vi "MTIF_Read_Simple.vi"(8 "error in":errorcluster, 9 "Input Parameters":T2={"Drop Bits"=3, "Output Files?"=TRUE, "STD Threshold Ratio for Start"=1.2, "STD Threshold Ratio for Stop"=1.1, "Output Image Type"=0, "Timeout for Queue(ms)"=1000, "Output Queue?"=FALSE, "Output File Format"=enum."AVI", "Initial STD Threshold"=12.0, "Number of Buffered Frames"=150, "Centroid Distence Threshold"=1.0} {"Output Image Type" items=["Grayscale (U8)", "Grayscale (I16)", "Grayscale (SGL)", "Complex (CSG)", "RGB (U32)", "HSL (U32)", "RGB (U64)", "Grayscale (U16)"]}, 10 "File Name (.mtif)":string="t8", 11 "Folder Path":path=path "X:/Zebrafish_VR_Data") -> (0 "error out":errorcluster, 2 "U8 Array Queue Out":refnum<queue>, 3 "U16 Array Queue Out":refnum<queue>)   [LabVIEW 2019]
uses:
  <vilib>/vision/NI_Vision_Development_Module.lvlib
panel:
  in  "Stop":bool
  out "Frame No.":i32=58
  out "Sequence No.":u16=3128
  out "Progress":dbl=1.0 format="%#.3f"
  out "Raw Image":T3(plugin-control)
  out "Frame Rate":dbl=550.0
  out "File ROI":T4={"Left"=0, "Top"=0, "Right"=639, "Bottom"=479, "Rotation"=0.0} {"Rotation" format="%.2f"; "Left" scale=0.0..1024.0; "Right" scale=0.0..1024.0}
  # "Max 2GB\nfor one AVI file!"
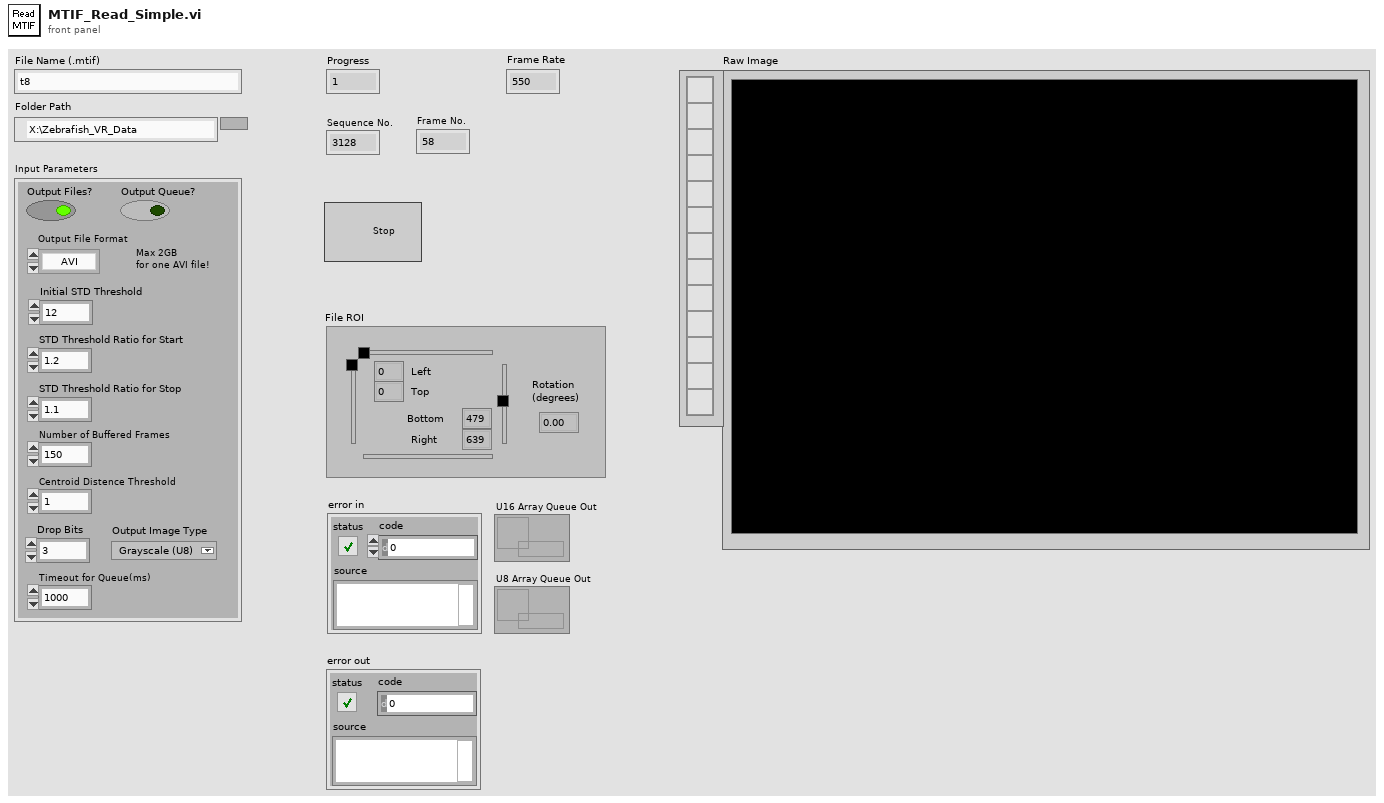
[diagram p1: front panel]
types:
  T1 = typedef "Image Type" = u32
  T2 = cluster{"Drop Bits":i8, "Output Files?":bool, "STD Threshold Ratio for Start":dbl, "STD Threshold Ratio for Stop":dbl, "Output Image Type":T1, "Timeout for Queue(ms)":u32, "Output Queue?":bool, "Output File Format":enum16{"TIFF", "AVI"}, "Initial STD Threshold":sgl, "Number of Buffered Frames":i32, "Centroid Distence Threshold":sgl}
  T3 = typedef "IMAQ Image.ctl" = refnum<image>
  T4 = typedef "IMAQ Rectangle" = cluster{"Left":i32, "Top":i32, "Right":i32, "Bottom":i32, "Rotation":dbl}
  T5 = enum16{"big-endian, network order", "native, host order", "little-endian"}
  T6 = enum16{"open", "replace", "create", "open or create", "replace or create", "replace or create with confirmation"}
  T7 = cluster{"[0]":i32, "[1]":i32, "[2]":i32, "[3]":i32}
  T8 = typedef "IMAQ AVI2 Refnum.ctl" = refnum<k20>
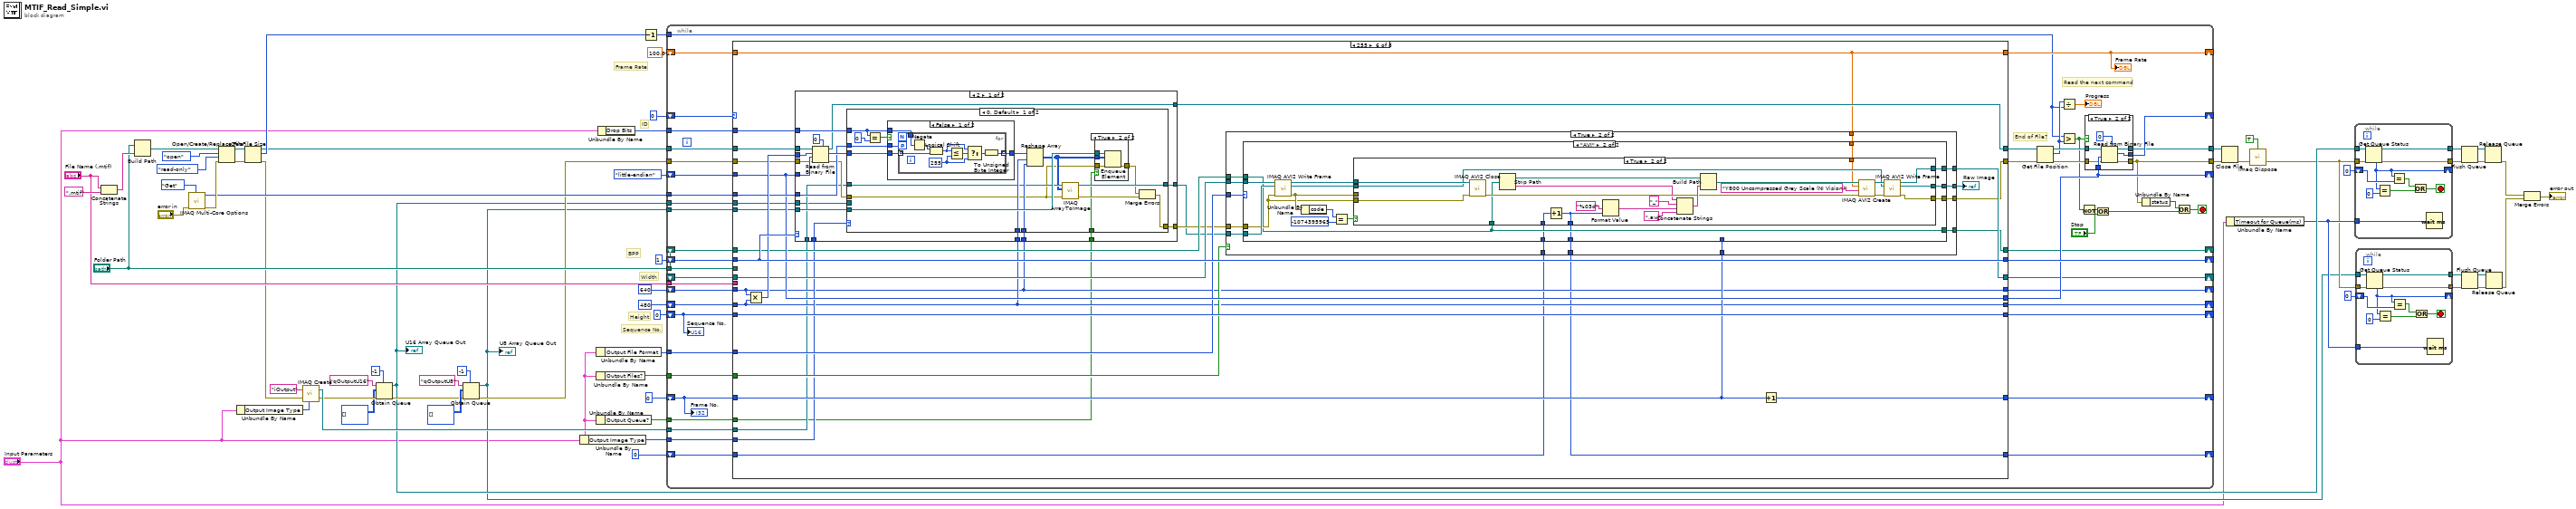
[diagram p0: block diagram]
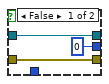
[diagram p2: hidden frame]
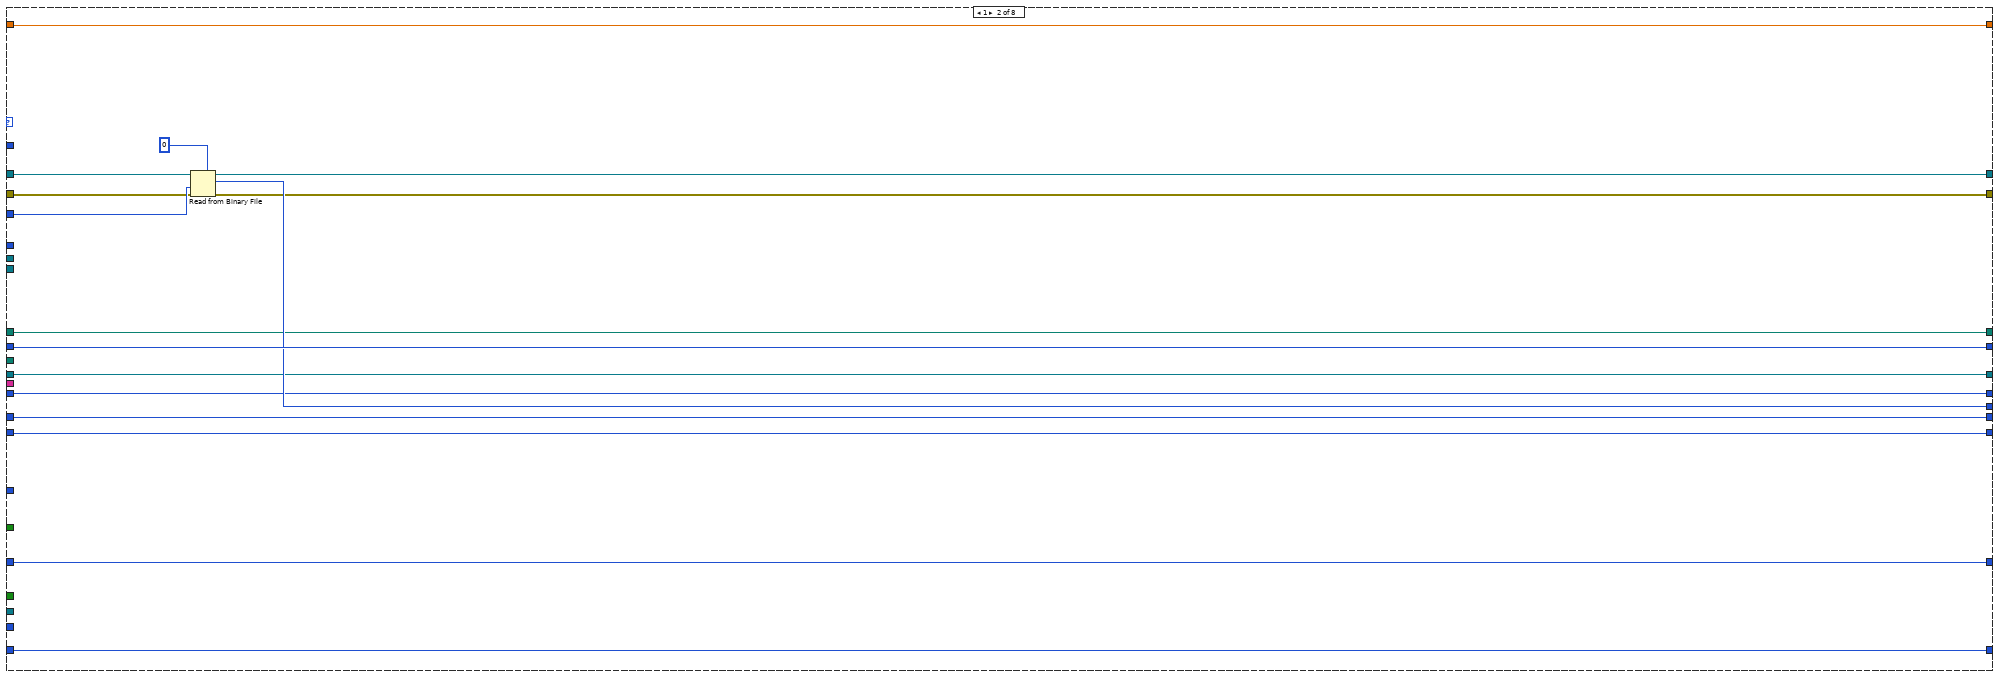
[diagram p4: hidden frame]
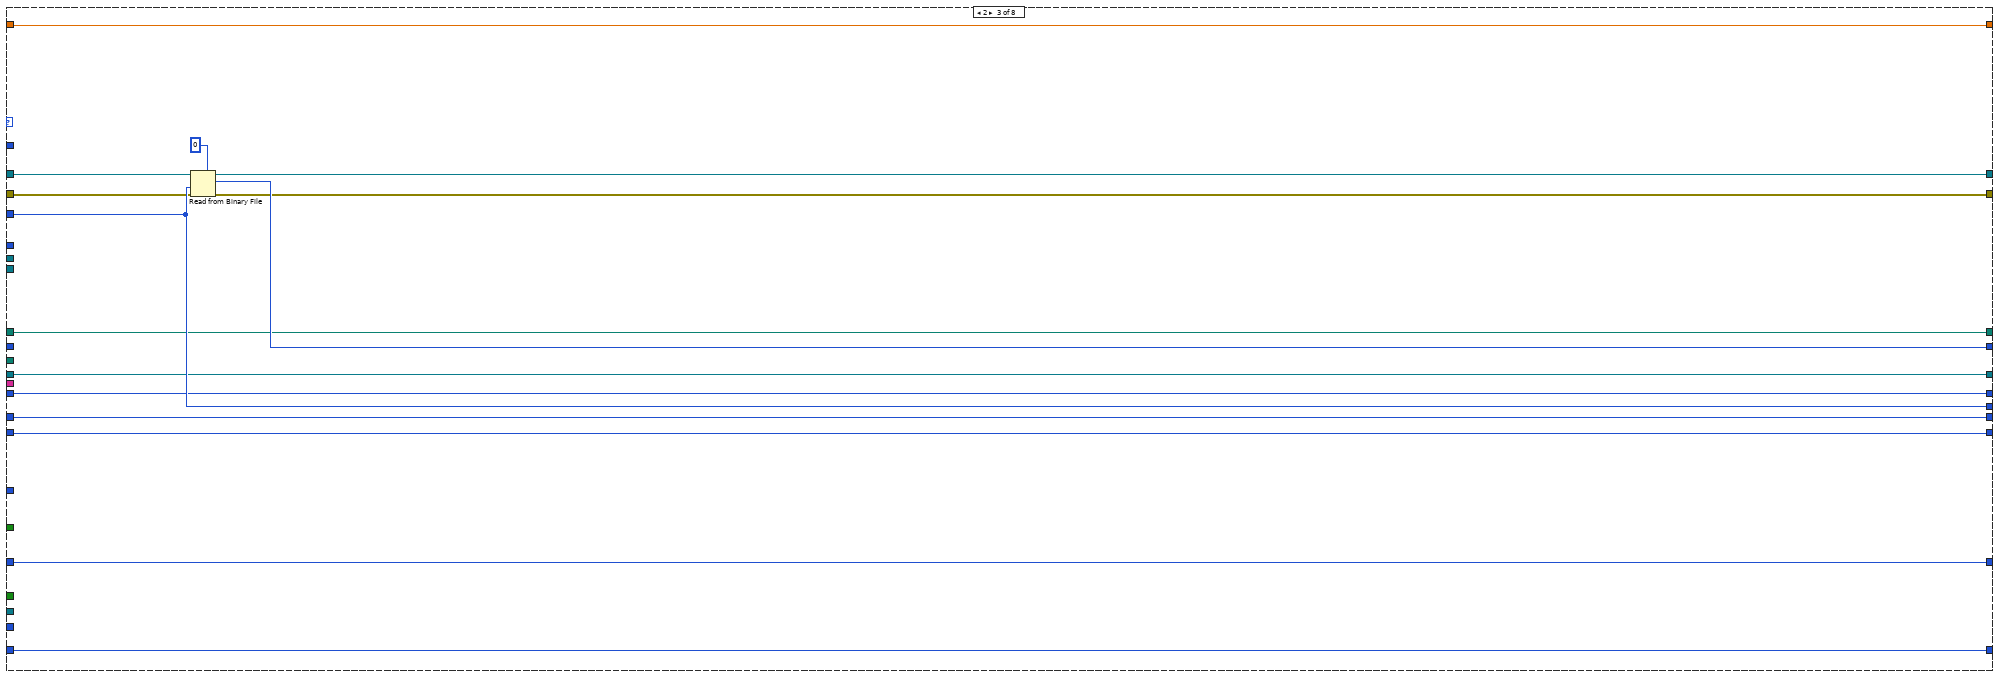
[diagram p5: hidden frame]
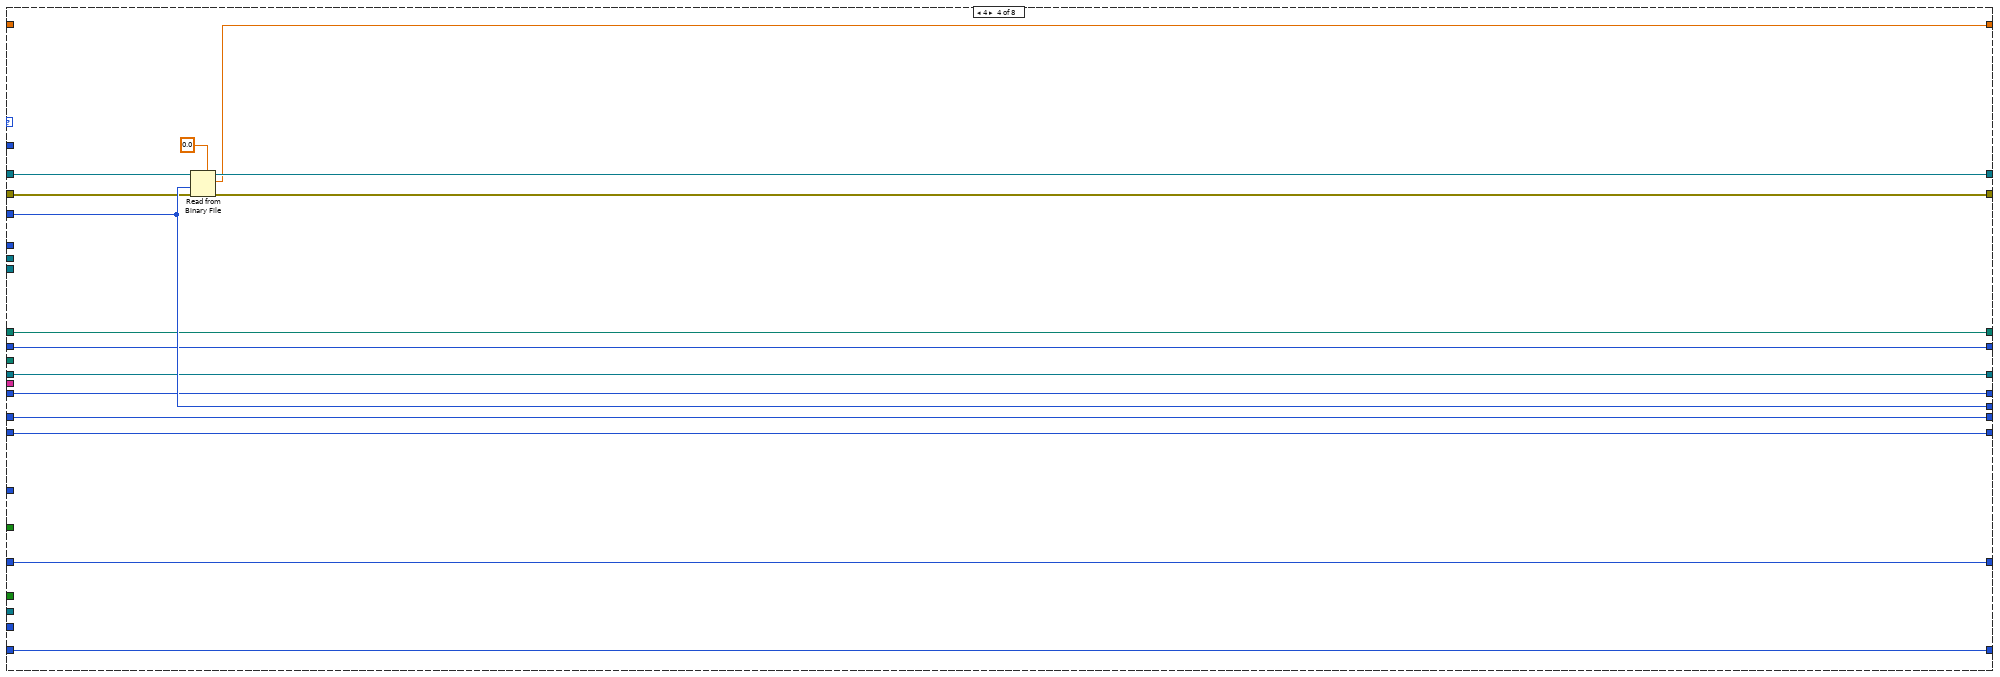
[diagram p6: hidden frame]
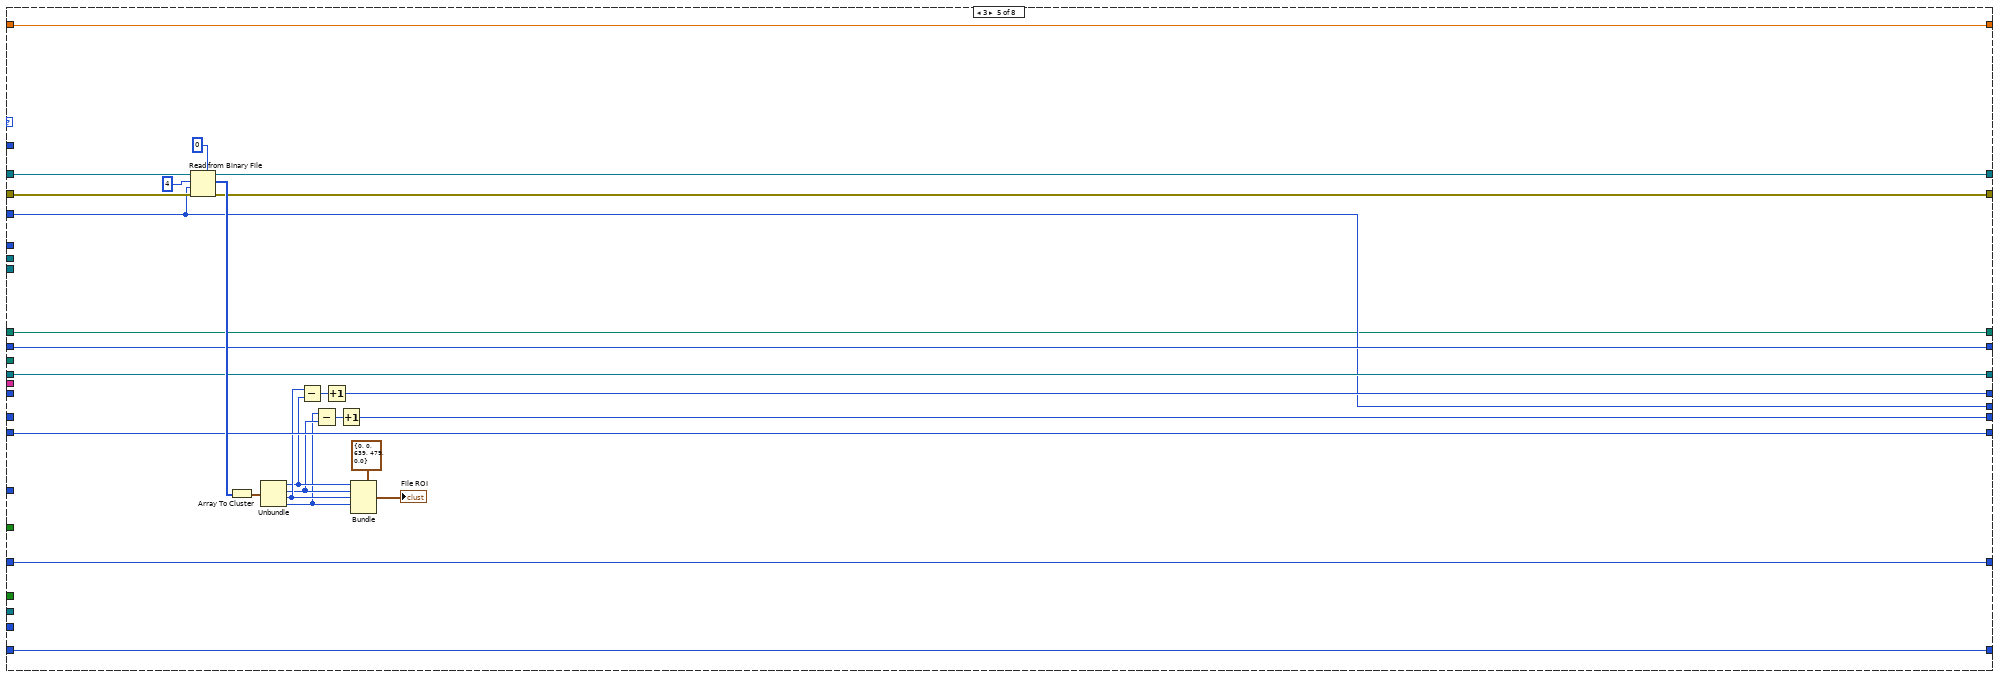
[diagram p7: hidden frame]
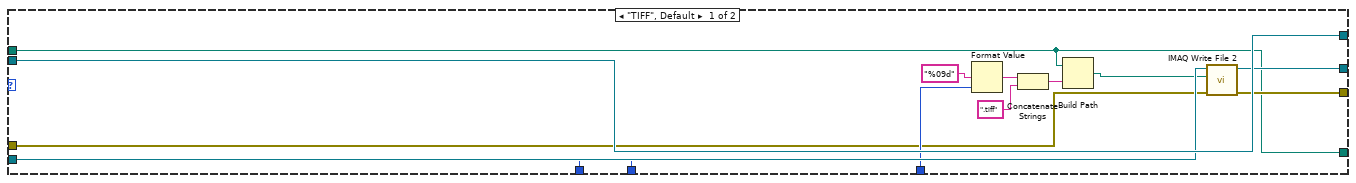
[diagram p9: hidden frame]
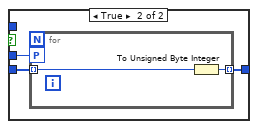
[diagram p11: hidden frame]
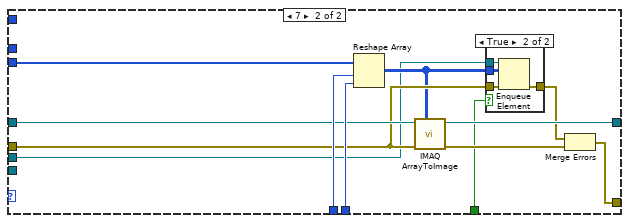
[diagram p13: hidden frame]
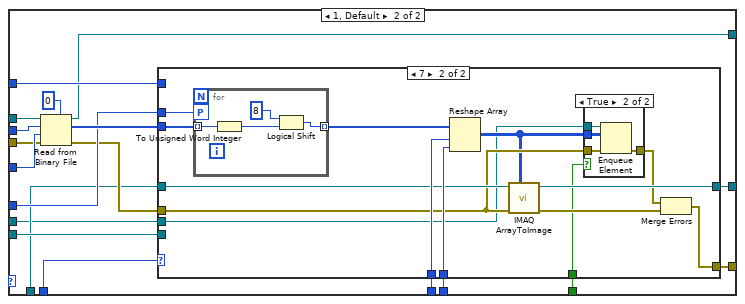
[diagram p15: hidden frame]
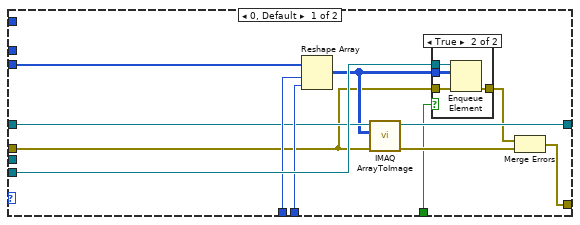
[diagram p16: hidden frame]
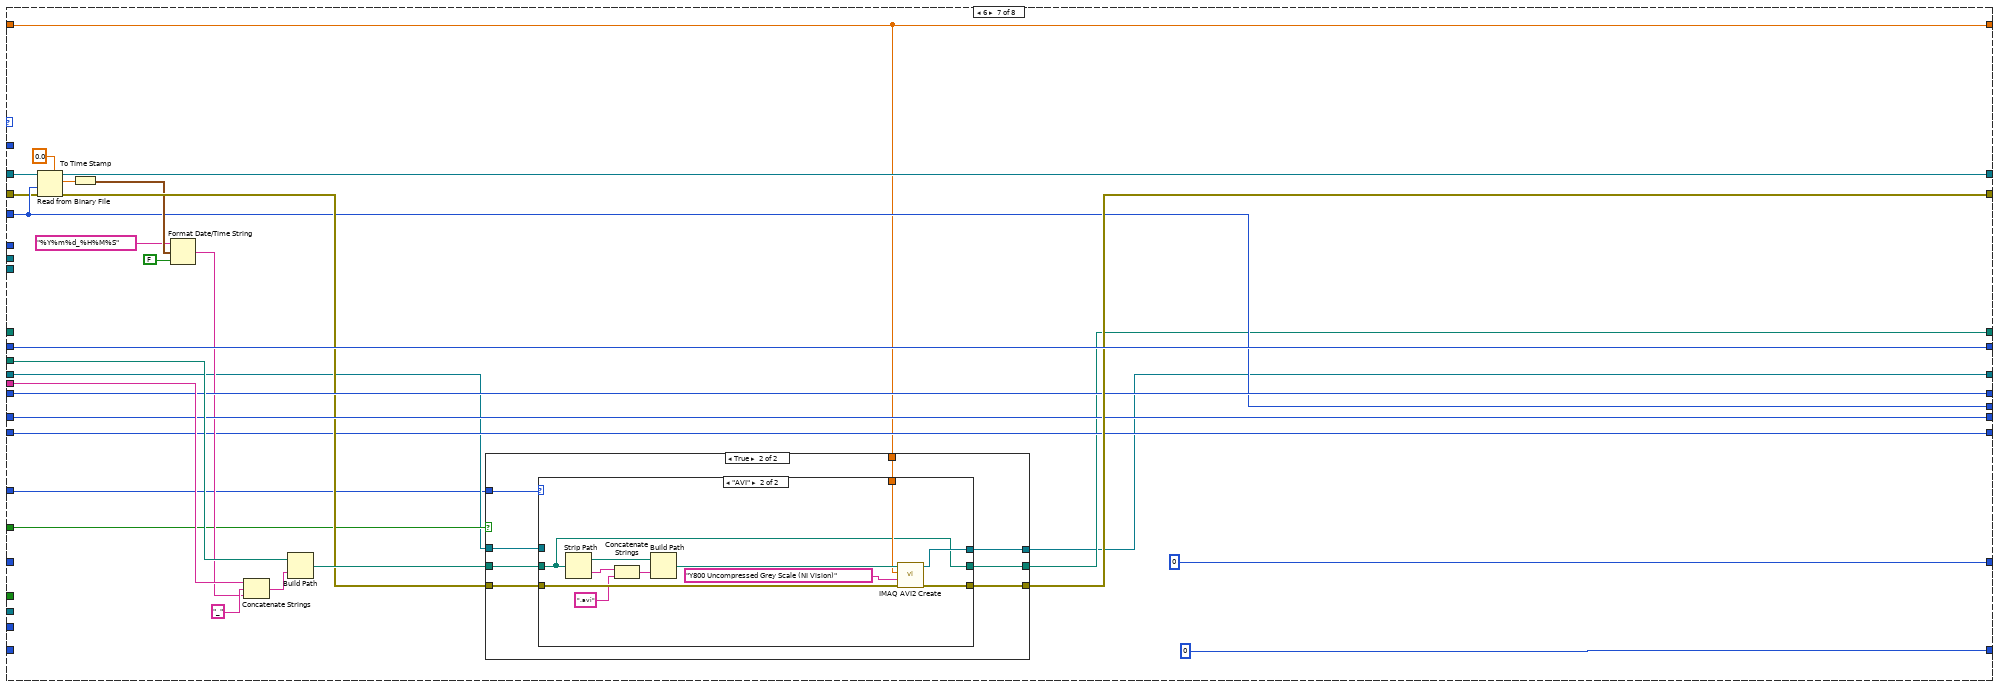
[diagram p19: hidden frame]
diagram:
  # "Sequence No."
  # "Height"
  # "Width"
  # "BPP"
  # "ID"
  # "Frame Rate"
  n1 = Concatenate Strings("File Name (.mtif)", ".mtif" ("string")) -> (w62:string)
  n2 = Build Path(base path="Folder Path", name or relative path=w62) -> (appended path=w58:path)
  n3 = call "IMAQ Multi-Core Options"("Get/Set Number of Cores (Get)"=enum32{"Get", "Set", "Set Max Available"}."Get", "error in (no error)"="error in") -> ("error out"=w48:errorcluster, "Cores Utilized"=w47:u32)  [unwired: 8 in]
  n4 = Open/Create/Replace File(file path (use dialog)=w58, error in=w48, operation (0:open)=T6."open", access (0:read/write)=enum16{"read/write", "read-only", "write-only"}."read-only") -> (refnum out=w53:refnum<file>, error out=w54:errorcluster)  [unwired: 2 in, 1 out]
  n5 = Unbundle By Name("Input Parameters") -> ("Output Image Type"=w27:T1)
  n6 = Get File Size(file=w53, error in=w54) -> (refnum out=w44:refnum<file>, size (in bytes)=w52:i64, 0:w21:errorcluster)
  n7 = call "IMAQ Create"("Image Name"="iOutput", "Image Type"=w27, "error in (no error)"=w21) -> ("New Image"=w26:T3, "error out"=w23:errorcluster)  [unwired: 2 in]
  n8 = Obtain Queue(max queue size (-1, unlimited)=-1, name (unnamed)="qOutputU16", element data type=u16[][] [], error in (no error)=w23) -> (queue out=w14:refnum<queue>, error out=w17:errorcluster)  [unwired: 1 in, 1 out]
  "U16 Array Queue Out" <- w14
  n9 = Obtain Queue(max queue size (-1, unlimited)=-1, name (unnamed)="qOutputU8", element data type=u8[][] [], error in (no error)=w17) -> (queue out=w3:refnum<queue>, error out=w16:errorcluster)  [unwired: 1 in, 1 out]
  "U8 Array Queue Out" <- w3
  n10 = Unbundle By Name("Input Parameters") -> ("Output Image Type"=w24:T1)
  n11 = Unbundle By Name("Input Parameters") -> ("Output File Format"=w30:enum16{"TIFF", "AVI"})
  n12 = Unbundle By Name("Input Parameters") -> ("Output Files?"=w33:bool)
  n13 = Unbundle By Name("Input Parameters") -> ("Output Queue?"=w32:bool)
  n14 = Unbundle By Name("Input Parameters") -> ("Drop Bits"=w31:i8)
  n15 = Decrement(x=w52) -> (x-1=w51:i64)
  n16 = while {
    shift-right: [w108] -> _
    shift-left: u8 0 -> [w115]
    shift-right: [w113] -> _
    shift-left: u8 1 -> [w114]
    tunnel: w44 -> [w112]
    shift-right: [w110] -> _
    shift-left: T5."little-endian" ("Byte Order") -> [w111]
    tunnel: w16 -> [w109]
    tunnel: [w69] -> w43
    shift-right: [w106] -> _
    shift-left: 100.0 -> [w107]
    shift-right: [w100] -> _
    shift-left: u16 0 -> [w105]
    shift-right: [w102] -> _
    shift-left: _ -> [w101]
    tunnel: w51 -> [w86]
    shift-right: [w94] -> _
    shift-left: 640 -> [w92]
    shift-right: [w93] -> _
    shift-left: 480 -> [w91]
    tunnel: w31 -> [w90]
    tunnel: w47 -> [w89]
    tunnel: w33 -> [w88]
    tunnel: [w84] -> w42
    tunnel: "Folder Path" -> [w104]
    tunnel: w14 -> [w83]
    tunnel: w32 -> [w82]
    tunnel: w30 -> [w81]
    tunnel: "File Name (.mtif)" -> [w103]
    shift-right: [w79] -> _
    shift-left: "Folder Path" -> [w80]
    tunnel: w26 -> [w76]
    shift-right: [w74] -> _
    shift-left: 0 -> [w75]
    tunnel: w24 -> [w73]
    tunnel: w3 -> [w72]
    shift-right: [w66] -> _
    shift-left: 0 -> [w67]
    stop <- w71 stop-if-true
    # "Read the next command"
    # "End of File?"
    n17 = case shown="255" w115 {
      tunnel: w111 -> [w137 w152 w167 w182 w187 w234 w459 w527]
      tunnel: [w137 w148 w167 w182 w187 w234 w459 w527] -> w110
      tunnel: w114 -> [w136 w151 _ w176 w199 w238 w476 w523]
      tunnel: [w136 w151 w164 w176 w199 w238 w476 w523] -> w113
      tunnel: w112 -> [w135 w150 w165 w180 w207 w240 w467 w525]
      tunnel: w109 -> [w134 w149 w166 w181 w208 w226 w449 w514]
      tunnel: [w134 w147 w163 w179 w185 w214 w471 w531] -> w98
      tunnel: [w135 w146 w162 w178 w206 w233 w466 w524] -> w99
      tunnel: [w133 w145 w161 w177 w200 w210 w450 w517] -> w106
      tunnel: w107 -> [w133 w145 w161 _ w200 w210 w450 w517]
      tunnel: w105 -> [w131 w143 w159 w174 w197 w239 w456 w521]
      tunnel: w104 -> [_ _ _ _ _ _ w474 _]
      tunnel: w103 -> [_ _ _ _ _ _ w473 _]
      tunnel: [w132 w144 w160 w175 w198 w231 w451 w518] -> w102
      tunnel: w101 -> [w132 w144 w160 w175 w198 w232 w453 w518]
      tunnel: [w131 w143 w159 w174 w197 w239 w456 w520] -> w100
      tunnel: [w130 w142 w158 w173 w190 w218 w469 w529] -> w94
      tunnel: [w129 w141 w157 w172 w189 w219 w470 w530] -> w93
      tunnel: w92 -> [w130 w142 w158 w173 _ w218 w469 w529]
      tunnel: w91 -> [w129 w141 w157 w172 _ w219 w470 w530]
      tunnel: w90 -> [_ _ _ _ _ w237 _ _]
      tunnel: w89 -> [_ _ _ _ _ w235 _ _]
      tunnel: w88 -> [_ _ _ _ _ w224 w458 w515]
      tunnel: w75 -> [w128 w140 w156 w171 w188 w225 _ w522]
      tunnel: [w128 w140 w156 w171 w188 w230 0 w522] -> w74
      tunnel: w83 -> [_ _ _ _ _ w216 _ _]
      tunnel: w82 -> [_ _ _ _ _ w213 _ _]
      tunnel: w81 -> [_ _ _ _ _ w229 w452 w519]
      tunnel: w80 -> [w127 w139 w155 w170 w186 w228 _ w516]
      tunnel: [w127 w139 w155 w170 w186 w227 w454 w516] -> w79
      tunnel: w76 -> [_ _ _ _ _ w217 _ _]
      tunnel: w73 -> [_ _ _ _ _ w221 _ _]
      tunnel: w72 -> [_ _ _ _ _ w220 _ _]
      tunnel: w67 -> [w126 w138 w154 w169 w184 w212 _ w513]
      tunnel: [w126 w138 w154 w169 w184 w211 0 w513] -> w66
      frame 0, Default {
      }
      frame 1 {
        n18 = Read from Binary File(5:u8 0, 8:w149, 9:w152, 11:w150) -> (0:w147:errorcluster, 2:w148:u8, 3:w146:refnum<file>)  [unwired: 2 in, 1 out]
      }
      frame 2 {
        n19 = Read from Binary File(5:u8 0, 8:w166, 9:w167, 11:w165) -> (0:w163:errorcluster, 2:w164:u8, 3:w162:refnum<file>)  [unwired: 2 in, 1 out]
      }
      frame 4 {
        n20 = Read from Binary File(5:0.0, 8:w181, 9:w182, 11:w180) -> (0:w179:errorcluster, 2:w177:dbl, 3:w178:refnum<file>)  [unwired: 2 in, 1 out]
      }
      frame 3 {
        n21 = Read from Binary File(5:0, 8:w208, 9:w187, 10:4 ("count (1)"), 11:w207) -> (0:w185:errorcluster, 2:w204:i32[], 3:w206:refnum<file>)  [unwired: 1 in, 1 out]
        n22 = Array To Cluster(array=w204) -> (cluster=w203:T7)
        n23 = Unbundle(w203) -> ("[0]"=w193:i32, "[1]"=w192:i32, "[2]"=w194:i32, "[3]"=w191:i32)
        n24 = Subtract(x=w194, y=w193) -> (x-y=w195:i32)
        n25 = Subtract(x=w191, y=w192) -> (x-y=w196:i32)
        n26 = Increment(x=w195) -> (x+1=w190:i32)
        n27 = Increment(x=w196) -> (x+1=w189:i32)
        n28 = Bundle(cluster=T4 {"Left"=0, "Top"=0, "Right"=639, "Bottom"=479, "Rotation"=0.0} ("Actual ROI"), "Left"=w193, "Top"=w192, "Right"=w194, "Bottom"=w191) -> (→"File ROI":T4)  [unwired: 1 in]
      }
      frame 255 {
        n29 = Multiply(x=w218, y=w219) -> (x*y=w236:i32)
        n30 = case shown="2" w238 {
          tunnel: w234 -> [w331 w406]
          tunnel: w226 -> [w330 w405]
          tunnel: w240 -> [w329 w404]
          tunnel: [w316 w391] -> w222
          tunnel: [w325 w400] -> w233
          tunnel: w237 -> [w327 w402]
          tunnel: w236 -> [w326 w401]
          tunnel: w235 -> [w324 w399]
          tunnel: w221 -> [w323 w398]
          tunnel: w220 -> [w322 w397]
          tunnel: w219 -> [w321 w396]
          tunnel: w218 -> [w320 w395]
          tunnel: w217 -> [w318 w393]
          tunnel: [w317 w392] -> w215
          tunnel: w216 -> [w315 w390]
          tunnel: w213 -> [w314 w389]
          frame 2 {
            n31 = Read from Binary File(5:u16 0, 8:w330, 9:w331, 10:w326, 11:w329) -> (0:w319:errorcluster, 2:w328:u16[], 3:w325:refnum<file>)  [unwired: 1 in, 1 out]
            n32 = case shown="0, Default" w323 {
              tunnel: w328 -> [w349 w375]
              tunnel: w327 -> [w335 _]
              tunnel: w324 -> [w348 _]
              tunnel: w322 -> [w347 _]
              tunnel: w321 -> [w345 w383]
              tunnel: w320 -> [w344 w382]
              tunnel: w319 -> [w341 w380]
              tunnel: w318 -> [w343 w381]
              tunnel: [w340 w379] -> w317
              tunnel: [w337 w376] -> w316
              tunnel: w315 -> [_ w373]
              tunnel: w314 -> [w336 w372]
              frame 0, Default {
                n33 = Equal?(x=w335, y=i8 0) -> (x = y?=w334:bool)
                n34 = case shown="False" w334 {
                  tunnel: w349 -> [w353 w364]
                  tunnel: w335 -> [w352 _]
                  tunnel: w348 -> [w351 w363]
                  tunnel: [w350 w362] -> w346
                  frame False {
                    n35 = for {
                      tunnel: w353 -> [w358] mode=indexing
                      tunnel: w352 -> [w356]
                      workers-P: w351 -> [_]
                      tunnel: [w354] -> w350 mode=indexing
                      w360 = u16 255 ("y")
                      n36 = Negate(x=w356) -> (-x=w357:i8)
                      n37 = Logical Shift(y=w357, x=w358) -> (x << y=w359:u16)
                      n38 = Less Or Equal?(x=w359, y=w360) -> (x <= y?=w361:bool)
                      n39 = Select(t=w359, s=w361, f=w360) -> (s? t:f=w355:u16)
                      n40 = To Unsigned Byte Integer(number=w355) -> (unsigned 8bit integer=w354:u8)
                    }
                  }
                  frame True {
                    n41 = for {
                      tunnel: w364 -> [w365] mode=indexing
                      workers-P: w363 -> [_]
                      tunnel: [w366] -> w362 mode=indexing
                      n42 = To Unsigned Byte Integer(number=w365) -> (unsigned 8bit integer=w366:u8)
                    }
                  }
                }
                n43 = Reshape Array(w346, w345, w344) -> (w342:u8[][])
                n44 = call "IMAQ ArrayToImage"("error in (no error)"=w341, "Image Pixels (U8)"=w342, "Image"=w343) -> ("error out"=w338:errorcluster, "Image Out"=w340:T3)  [unwired: 7 in]
                n45 = case shown="True" w336 {
                  tunnel: w347 -> [_ w371]
                  tunnel: w342 -> [_ w370]
                  tunnel: w341 -> [w367 w369]
                  tunnel: [w367 w368] -> w339
                  frame False {
                  }
                  frame True {
                    n46 = Enqueue Element(queue=w371, element=w370, error in (no error)=w369) -> (error out=w368:errorcluster)  [unwired: 1 in, 2 out]
                  }
                }
                n47 = Merge Errors(w339, w338) -> (w337:errorcluster)
              }
              frame 7 {
                n48 = Reshape Array(w375, w383, w382) -> (w374:u16[][])
                n49 = call "IMAQ ArrayToImage"("Image Pixels (U16)"=w374, "error in (no error)"=w380, "Image"=w381) -> ("error out"=w377:errorcluster, "Image Out"=w379:T3)  [unwired: 7 in]
                n50 = case shown="True" w372 {
                  tunnel: w380 -> [w384 w388]
                  tunnel: [w384 w387] -> w378
                  tunnel: w374 -> [_ w386]
                  tunnel: w373 -> [_ w385]
                  frame False {
                  }
                  frame True {
                    n51 = Enqueue Element(queue=w385, element=w386, error in (no error)=w388) -> (error out=w387:errorcluster)  [unwired: 1 in, 2 out]
                  }
                }
                n52 = Merge Errors(w378, w377) -> (w376:errorcluster)
              }
            }
          }
          frame 1, Default {
            n53 = Read from Binary File(5:u8 0, 8:w405, 9:w406, 10:w401, 11:w404) -> (0:w394:errorcluster, 2:w403:u8[], 3:w400:refnum<file>)  [unwired: 1 in, 1 out]
            n54 = case shown="7" w398 {
              tunnel: w403 -> [w409 w427]
              tunnel: w402 -> [_ _]
              tunnel: w399 -> [_ w428]
              tunnel: w397 -> [w419 _]
              tunnel: w396 -> [w418 w438]
              tunnel: w395 -> [w417 w437]
              tunnel: w394 -> [w414 w435]
              tunnel: w393 -> [w416 w436]
              tunnel: [w413 w434] -> w392
              tunnel: [w410 w431] -> w391
              tunnel: w390 -> [_ w429]
              tunnel: w389 -> [w408 w425]
              frame 0, Default {
                n55 = Reshape Array(w409, w418, w417) -> (w415:u8[][])
                n56 = call "IMAQ ArrayToImage"("error in (no error)"=w414, "Image Pixels (U8)"=w415, "Image"=w416) -> ("error out"=w411:errorcluster, "Image Out"=w413:T3)  [unwired: 7 in]
                n57 = case shown="True" w408 {
                  tunnel: w419 -> [_ w424]
                  tunnel: w415 -> [_ w423]
                  tunnel: w414 -> [w420 w422]
                  tunnel: [w420 w421] -> w412
                  frame False {
                  }
                  frame True {
                    n58 = Enqueue Element(queue=w424, element=w423, error in (no error)=w422) -> (error out=w421:errorcluster)  [unwired: 1 in, 2 out]
                  }
                }
                n59 = Merge Errors(w412, w411) -> (w410:errorcluster)
              }
              frame 7 {
                n60 = for {
                  tunnel: w427 -> [w446] mode=indexing
                  workers-P: w428 -> [_]
                  tunnel: [w444] -> w426 mode=indexing
                  n61 = To Unsigned Word Integer(number=w446) -> (unsigned 16bit integer=w445:u16)
                  n62 = Logical Shift(y=i16 8, x=w445) -> (x << y=w444:u16)
                }
                n63 = Reshape Array(w426, w438, w437) -> (w430:u16[][])
                n64 = call "IMAQ ArrayToImage"("Image Pixels (U16)"=w430, "error in (no error)"=w435, "Image"=w436) -> ("error out"=w432:errorcluster, "Image Out"=w434:T3)  [unwired: 7 in]
                n65 = case shown="True" w425 {
                  tunnel: w435 -> [w439 w443]
                  tunnel: [w439 w442] -> w433
                  tunnel: w430 -> [_ w441]
                  tunnel: w429 -> [_ w440]
                  frame False {
                  }
                  frame True {
                    n66 = Enqueue Element(queue=w440, element=w441, error in (no error)=w443) -> (error out=w442:errorcluster)  [unwired: 1 in, 2 out]
                  }
                }
                n67 = Merge Errors(w433, w432) -> (w431:errorcluster)
              }
            }
          }
        }
        n68 = case shown="True" w224 {
          tunnel: w222 -> [w245 w250]
          tunnel: w215 -> [w243 w249]
          tunnel: [w245 w258] -> w214
          tunnel: w232 -> [w244 w255]
          tunnel: [w244 w257] -> w231
          tunnel: w228 -> [w242 w256]
          tunnel: w229 -> [_ w254]
          tunnel: [w243 w253] -> w223
          tunnel: [w242 w252] -> w227
          tunnel: w225 -> [_ w251]
          tunnel: w212 -> [w241 w248]
          tunnel: [w241 w247] -> w211
          tunnel: w210 -> [_ w246]
          frame False {
          }
          frame True {
            n69 = case shown="\"AVI\"" w254 {
              tunnel: [w270 w278] -> w258
              tunnel: [w271 w279] -> w257
              tunnel: w250 -> [w260 w276]
              tunnel: w256 -> [w265 w275]
              tunnel: w255 -> [w271 w287]
              tunnel: w249 -> [w269 w286]
              tunnel: [w268 w277] -> w253
              tunnel: [w265 w275] -> w252
              tunnel: w251 -> [w266 _]
              tunnel: w248 -> [w259 w274]
              tunnel: [w259 w273] -> w247
              tunnel: w246 -> [_ w272]
              frame "TIFF", Default {
                n70 = Format Value(format string="%09d", value (0)=w266) -> (output string=w263:string)  [unwired: 1 in]
                n71 = Concatenate Strings(w263, ".tiff" ("string")) -> (w262:string)
                n72 = Build Path(base path=w265, name or relative path=w262) -> (appended path=w261:path)
                n73 = call-poly "IMAQ Write File 2"("error in (no error)"=w260, "File Path"=w261, "Image"=w269) -> ("error out"=w270:errorcluster, "Image Out (duplicate)"=w268:T3)  [unwired: 7 in]
              }
              frame "AVI" {
                n74 = call "IMAQ AVI2 Write Frame"("error in (no error)"=w276, "Image"=w286, "AVI Refnum"=w287) -> ("error out"=w281:errorcluster, "Image Out (duplicate)"=w280:T3, "AVI Refnum (duplicate)"=w282:T8)  [unwired: 6 in]
                n75 = Unbundle By Name(w281) -> ("code"=w285:i32)
                n76 = Equal?(x=w285, y=-1074395965) -> (x = y?=w283:bool)
                n77 = case shown="True" w283 {
                  tunnel: w282 -> [w291 w313]
                  tunnel: w281 -> [w290 _]
                  tunnel: w280 -> [w289 w304]
                  tunnel: [w291 w301] -> w279
                  tunnel: [w290 w302] -> w278
                  tunnel: [w289 w300] -> w277
                  tunnel: w276 -> [_ w312]
                  tunnel: w275 -> [_ w299]
                  tunnel: w274 -> [w288 w294]
                  tunnel: [w288 w293] -> w273
                  tunnel: w272 -> [_ w292]
                  frame False {
                  }
                  frame True {
                    n78 = call "IMAQ AVI2 Close"("error in (no error)"=w312, "AVI Refnum"=w313) -> ("error out"=w303:errorcluster)  [unwired: 9 in]
                    n79 = Strip Path(path=w299) -> (stripped path=w310:path, name=w298:string)
                    n80 = Increment(x=w294) -> (x+1=w293:i32)
                    n81 = Format Value(format string="%03d", value (0)=w293) -> (output string=w295:string)  [unwired: 1 in]
                    n82 = Concatenate Strings(w298, "_" ("string"), w295, ".avi" ("string")) -> (w308:string)
                    n83 = Build Path(base path=w310, name or relative path=w308) -> (appended path=w307:path)
                    n84 = call "IMAQ AVI2 Create"("error in (no error)"=w303, "Codec"="Y800 Uncompressed Grey Scale (NI Vision)", "Frames Per Second"=w292, "AVI Path"=w307) -> ("error out"=w306:errorcluster, "AVI Refnum"=w305:T8)  [unwired: 6 in]
                    n85 = call "IMAQ AVI2 Write Frame"("error in (no error)"=w306, "Image"=w304, "AVI Refnum"=w305) -> ("error out"=w302:errorcluster, "Image Out (duplicate)"=w300:T3, "AVI Refnum (duplicate)"=w301:T8)  [unwired: 6 in]
                  }
                }
              }
            }
          }
        }
        "Raw Image" <- w223
        n86 = Increment(x=w225) -> (x+1=w230:i32)
      }
      frame 6 {
        n87 = Read from Binary File(5:0.0, 8:w449, 9:w459, 11:w467) -> (0:w465:errorcluster, 2:w464:dbl, 3:w466:refnum<file>)  [unwired: 2 in, 1 out]
        n88 = To Time Stamp(1:w464) -> (0:w462:timestamp)
        n89 = Format Date/Time String(time format string (%c)="%Y%m%d_%H%M%S", seconds (now)=w462, UTC format=FALSE) -> (date/time string=w463:string)
        n90 = Concatenate Strings(w473, "_", w463) -> (w455:string)
        n91 = Build Path(base path=w474, name or relative path=w455) -> (appended path=w475:path)
        n92 = case shown="True" w458 {
          tunnel: w475 -> [w478 w487]
          tunnel: [w479 w485] -> w471
          tunnel: w465 -> [w479 w486]
          tunnel: [w478 w484] -> w454
          tunnel: w453 -> [w477 w481]
          tunnel: w452 -> [_ w483]
          tunnel: [w477 w482] -> w451
          tunnel: w450 -> [_ w480]
          frame False {
          }
          frame True {
            n93 = case shown="\"AVI\"" w483 {
              tunnel: w487 -> [w495 w504]
              tunnel: w486 -> [w494 w512]
              tunnel: [w490 w508] -> w485
              tunnel: [w489 w504] -> w484
              tunnel: [w488 w510] -> w482
              tunnel: w481 -> [w488 _]
              tunnel: w480 -> [_ w509]
              frame "TIFF", Default {
                n94 = call <vilib>:"Check if File or Folder Exists.vi"("error in (no error)"=w494, "path"=w495) -> ("error out"=w491:errorcluster, "file or folder exists?"=w493:bool, "dup path"=w492:path)  [unwired: 7 in]
                n95 = case shown="False" w493 {
                  tunnel: w492 -> [w499 w500]
                  tunnel: w491 -> [w498 w501]
                  tunnel: [w497 w501] -> w490
                  tunnel: [w496 w500] -> w489
                  frame False {
                    n96 = Create Folder(path (use dialog)=w499, error in=w498) -> (created path=w496:path, error out=w497:errorcluster)  [unwired: 1 in, 1 out]
                  }
                  frame True {
                  }
                }
              }
              frame "AVI" {
                n97 = Strip Path(path=w504) -> (stripped path=w503:path, name=w505:string)
                n98 = Concatenate Strings(w505, ".avi" ("string")) -> (w507:string)
                n99 = Build Path(base path=w503, name or relative path=w507) -> (appended path=w511:path)
                n100 = call "IMAQ AVI2 Create"("error in (no error)"=w512, "Codec"="Y800 Uncompressed Grey Scale (NI Vision)", "Frames Per Second"=w509, "AVI Path"=w511) -> ("error out"=w508:errorcluster, "AVI Refnum"=w510:T8)  [unwired: 6 in]
              }
            }
          }
        }
      }
      frame 7 {
        n101 = Increment(x=w521) -> (x+1=w520:u16)
        n102 = Read from Binary File(5:0.0, 8:w514, 9:w527, 11:w525) -> (0:w526:errorcluster, 3:w524:refnum<file>)  [unwired: 2 in, 2 out]
        n103 = case shown="True" w515 {
          tunnel: [w532 w536] -> w531
          tunnel: w526 -> [w532 w535]
          tunnel: w519 -> [_ w534]
          tunnel: w518 -> [_ w533]
          frame False {
          }
          frame True {
            n104 = case shown="\"AVI\"" w534 {
              tunnel: [w537 w540] -> w536
              tunnel: w535 -> [w537 w539]
              tunnel: w533 -> [_ w538]
              frame "TIFF", Default {
              }
              frame "AVI" {
                n105 = call "IMAQ AVI2 Close"("error in (no error)"=w539, "AVI Refnum"=w538) -> ("error out"=w540:errorcluster)  [unwired: 9 in]
              }
            }
          }
        }
      }
    }
    "Frame Rate" <- w106
    n106 = Get File Position(4:w98, 7:w99) -> (0:w96:errorcluster, 2:w87:i64, 3:w97:refnum<file>)
    n107 = Divide(x=w87, y=w86) -> (x/y=→"Progress":dbl)
    n108 = Greater?(x=w86, y=w87) -> (0:w95:bool)
    n109 = Not(x=w95) -> (.not. x?=w78:bool)
    n110 = case shown="True" w95 {
      tunnel: w110 -> [_ w124]
      tunnel: [u8 0 w123] -> w108
      tunnel: [w117 w122] -> w69
      tunnel: w97 -> [w116 w121]
      tunnel: w96 -> [w117 w120]
      tunnel: [w116 w119] -> w84
      frame False {
      }
      frame True {
        n111 = Read from Binary File(5:u8 0, 8:w120, 9:w124, 11:w121) -> (0:w122:errorcluster, 2:w123:u8, 3:w119:refnum<file>)  [unwired: 2 in, 1 out]
      }
    }
    n112 = Or(x=w78, y="Stop") -> (x .or. y?=w70:bool)
    n113 = Unbundle By Name(w69) -> ("status"=w68:bool)
    n114 = Or(x=w68, y=w70) -> (x .or. y?=w71:bool)
    "Sequence No." <- w105
    "Frame No." <- w75
  }
  n115 = Close File(refnum=w42, error in=w43) -> (error out=w39:errorcluster)  [unwired: 1 out]
  n116 = Unbundle By Name("Input Parameters") -> ("Timeout for Queue(ms)"=w8:u32)
  n117 = call "Imaq Dispose"("All Images? (No)"=TRUE, "error in (no error)"=w39) -> ("error out"=w7:errorcluster)  [unwired: 4 in]
  n118 = while {
    tunnel: w14 -> [w551]
    tunnel: w7 -> [w550]
    tunnel: [w549] -> w37
    tunnel: [w548] -> w38
    shift-right: [w545] -> _
    shift-left: 0 ("# elements in queue") -> [w546]
    tunnel: w8 -> [w541]
    stop <- w542 stop-if-true
    n119 = Get Queue Status(queue=w551, error in (no error)=w550) -> (queue out=w548:refnum<queue>, error out=w549:errorcluster, # elements in queue=w545:i32)  [unwired: 1 in, 5 out]
    n120 = Equal?(x=w545, y=0) -> (x = y?=w543:bool)
    n121 = Equal?(x=w545, y=w546) -> (x = y?=w544:bool)
    n122 = Or(x=w544, y=w543) -> (x .or. y?=w542:bool)
    n123 = Wait (ms)(milliseconds to wait=w541) -> ()  [unwired: 1 out]
  }
  n124 = while {
    tunnel: w3 -> [w562]
    tunnel: w7 -> [w561]
    tunnel: [w560] -> w12
    tunnel: [w559] -> w13
    shift-right: [w556] -> _
    shift-left: 0 ("# elements in queue") -> [w557]
    tunnel: w8 -> [w552]
    stop <- w553 stop-if-true
    n125 = Get Queue Status(queue=w562, error in (no error)=w561) -> (queue out=w559:refnum<queue>, error out=w560:errorcluster, # elements in queue=w556:i32)  [unwired: 1 in, 5 out]
    n126 = Equal?(x=w556, y=0) -> (x = y?=w554:bool)
    n127 = Equal?(x=w556, y=w557) -> (x = y?=w555:bool)
    n128 = Or(x=w555, y=w554) -> (x .or. y?=w553:bool)
    n129 = Wait (ms)(milliseconds to wait=w552) -> ()  [unwired: 1 out]
  }
  n130 = Flush Queue(queue=w38, error in (no error)=w37) -> (queue out=w35:refnum<queue>, error out=w36:errorcluster)  [unwired: 1 out]
  n131 = Flush Queue(queue=w13, error in (no error)=w12) -> (queue out=w10:refnum<queue>, error out=w11:errorcluster)  [unwired: 1 out]
  n132 = Release Queue(queue=w35, error in (no error)=w36) -> (error out=w6:errorcluster)  [unwired: 1 in, 2 out]
  n133 = Release Queue(queue=w10, error in (no error)=w11) -> (error out=w5:errorcluster)  [unwired: 1 in, 2 out]
  n134 = Merge Errors(w6, w5) -> (→"error out":errorcluster)
